vi "Table tes.vi"() -> ()   [LabVIEW 2025]
uses:
  Controls/Test Results/Results Table.ctl
panel:
  in  "Table Control 2":T1=[["Wear-in", "N/A", "N/A", "", "", "", "", ""], ["Drop-out", "N/A", "N/A", "", "", "", "", ""], ["Closing Response Time", "N/A", "N/A", "", "", "", "", ""], ["Pull-in", "N/A", "N/A", "", "", "", "", ""], ["Hold-in", "N/A", "N/A", "", "", "", "", ""], ["Opening Response Time", "N/A", "N/A", "", "", "", "", ""]]
  out "element":string
  in  "Table Control":string[][](table)
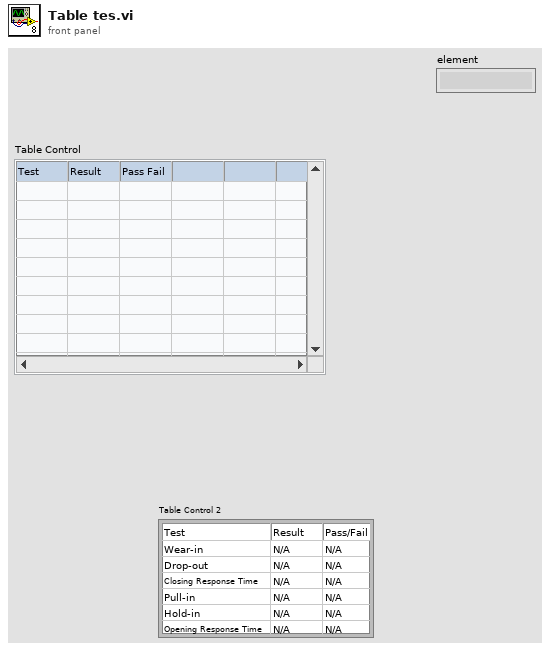
[diagram p1: front panel]
types:
  T1 = typedef "Results Table.ctl" = string[][]
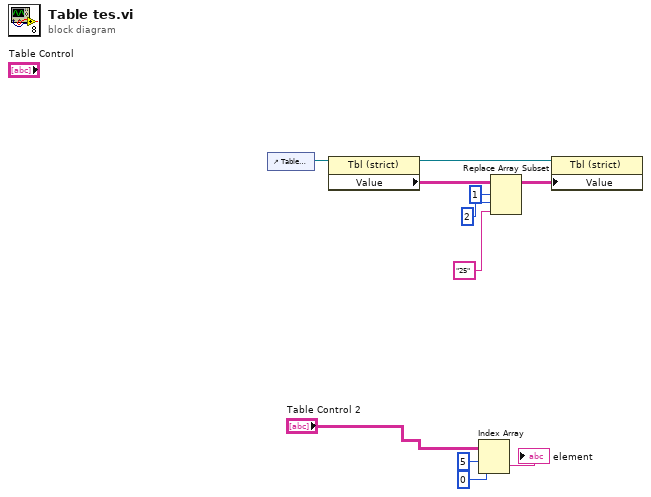
[diagram p0: block diagram]
diagram:
  n1 = control-ref of="Table Control"() -> (w11:refnum<vi>)
  n2 = property class="Tbl (strict)"(reference=w11) -> (reference out=w10:refnum<vi>, "Value"=w8:string[][])  [unwired: 1 in, 1 out]
  n3 = Index Array(array="Table Control 2", index (row)=5, index (col)=0 ("disabled index (col)")) -> (element=→"element":string)
  n4 = Replace Array Subset(array=w8, new element="25" ("new element/subarray"), index (row)=1, index (col)=2) -> (w9:string[][])
  n5 = property class="Tbl (strict)"(reference=w10, "Value"=w9) -> ()  [unwired: 1 in, 2 out]
